vi "XORFilter.vi"(0 "Image Src 1":T1, 1 "Filtered Image Dst 1":T1, 2 "Processed Image Dst 2":T1, 3 "Image Src 2":T1, 4 "Filtered Image Dst 2":T1, 5 "Processed Image Dst 2":T1, 7 "XOR Image Dst":T1, 9 "Threshold Range":cluster{"Lower value":sgl, "Upper value":sgl}={"Lower value"=240.0, "Upper value"=255.0} {"Upper value" format="%.2f"; "Lower value" format="%.2f"}) -> (14 "XOR Image Dst Out":T1, 15 "Image Dst 1 Out":T1, 16 "Image Dst 2 Out":T1)   [LabVIEW 2011]
uses:
  <vilib>/vision/Image Controls.llb/IMAQ Image.ctl
  <vilib>/vision/NI_Vision_Development_Module.lvlib
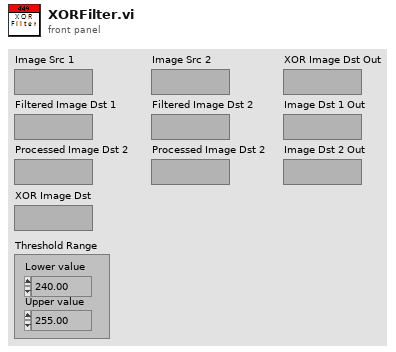
[diagram p1: front panel]
types:
  T1 = typedef "IMAQ Image.ctl" = refnum<image>
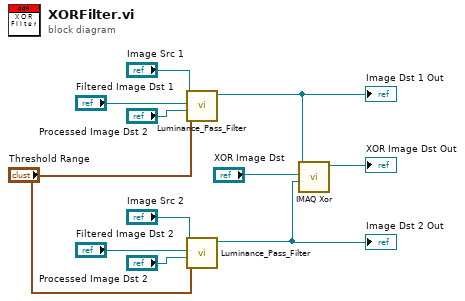
[diagram p0: block diagram]
diagram:
  n1 = call "Luminance_Pass_Filter.vi"("Threshold Range"="Threshold Range", "Processed Image Dst"="Processed Image Dst 2", "Filtered Image Dst"="Filtered Image Dst 1", "Image Src"="Image Src 1") -> ("Image Dst Out"=w2:T1)  [unwired: 7 in]
  "Image Dst 1 Out" <- w2
  n2 = call "Luminance_Pass_Filter.vi"("Threshold Range"="Threshold Range", "Processed Image Dst"="Processed Image Dst 2", "Filtered Image Dst"="Filtered Image Dst 2", "Image Src"="Image Src 2") -> ("Image Dst Out"=w3:T1)  [unwired: 7 in]
  "Image Dst 2 Out" <- w3
  n3 = call "IMAQ Xor"("Image Src B"=w3, "Image Dst"="XOR Image Dst", "Image Src A"=w2) -> ("Image Dst Out"=→"XOR Image Dst Out":T1)  [unwired: 7 in, 1 out]
